vi "DMM DCVM Immediate Trigger Delay.vi"() -> ()   [LabVIEW 2021]
uses:
  DMM_DC-RMS Voltage Measurement/Typedefs/Function Settings.ctl
  <instrlib>/niDMM/nidmm.llb/niDMM Resolution in Digits.ctl
  DMM_DC-RMS Voltage Measurement/Typedefs/Timing & Trigger Settings.ctl
  <instrlib>/niDMM/nidmm.llb/niDMM Trigger.ctl
  <instrlib>/niDMM/nidmm.llb/niDMM Slope.ctl
  DMM_DC-RMS Voltage Measurement/Typedefs/Measurement.ctl
  DMM Mixed Measurements/DMM Mixed Meas Typedefs/DMM Execution Settings.ctl
  Signal Voltage Generation/Typedefs/Signal Generation Settings.ctl
  Signal Voltage Generation/Typedefs/Generation Types.ctl
  Signal Voltage Generation/Typedefs/Single Tone Settings.ctl
  Signal Voltage Generation/Typedefs/Waveform Type.ctl
  Signal Voltage Generation/Typedefs/Tone Settings.ctl
  Common/Typedefs/Execution Options - Measure.ctl
  DMM_DC-RMS Voltage Measurement/DMM_DC-RMS Voltage Measurement.lvlib
  Signal Voltage Generation/DAQ_Signal Voltage Generation.lvlib
  DMM Mixed Measurements/DMM_Mixed Measurement.lvlib
panel:
  in  "Signal Generation Settings":T1={"Generation Type"=enum."Single Tone", "Generation Time (s)"=4.0, "Voltage Offset (v)"=0.0, "Single Tone Settings"={"Waveform Type"=enum."Sine Wave", "Frequency (Hz)"=100.0, "Amplitude (V)"=1.0, "Duty Cycle (%)"=50.0}, "Multi Tone Settings"=[]} {"Voltage Offset (v)" format="%.2p"; "Generation Time (s)" format="%.2p"; "Multi Tone Settings"."Amplitude (V)" format="%.2p"; "Multi Tone Settings"."Frequency (Hz)" format="%.2p"; "Single Tone Settings"."Duty Cycle (%)" format="%.2p"; "Single Tone Settings"."Amplitude (V)" format="%.2p"; "Single Tone Settings"."Frequency (Hz)" format="%.2p"}
  out "error out":errorcluster
  out "DMM Execution Settings":T6={"Absolute\nResolution"=2.4999999999999998e-05, "Input Resistance\n(Ohm)"=1000000.0, "Digits\nResolution"=5.5, "Range"=5.0, "Minimum\nFrequency (Hz)"=40.0, "Aperture\nTime (s)"=0.1, "Auto Range\nValue"=5.0, "Settle\nTime (s)"=1.0, "Function"=2} {"Function" items=["DC Volts"=1, "AC Volts"=2, "DC Current"=3, "AC Current"=4, "2-Wire Resistance"=5, "4-Wire Resistance"=101, "Frequency"=104, "Period"=105, "AC Volts DC Coupled"=1001, "Diode"=1002, "Waveform Voltage"=1003, "Waveform Current"=1004, "Capacitance"=1005, "Inductance"=1006, "Temperature"=108]; "Absolute\nResolution" format="%#_6p"; "Input Resistance\n(Ohm)" format="%#_6p"; "Range" format="%#_6p"; "Minimum\nFrequency (Hz)" format="%#_6p"; "Aperture\nTime (s)" format="%#_6p"; "Auto Range\nValue" format="%#_6p"; "Settle\nTime (s)" format="%#_6p"}
  out "Measurement":T7={"Measured Value"=0.7067715989184996, "Out of Range"=FALSE, "Unit"="V (ac)", "Measurement"="706.772mV (ac)"} {"Measured Value" format="%^#_9e"}
  in  "Timing and Trigger Settings":T8={"AC Min Frequency (Hz)"=40.0, "Aperture Time (s)"=-1.0, "Settle Time (s)"=-1.0, "Trigger Settings"={"Trigger Delay (sec)"=2.0, "Enable Trigger?"=TRUE, "Trigger Source"=enum."Immediate", "Slope"=enum."Rising Edge"}} {"Trigger Settings"."Trigger Delay (sec)" format="%.4f"; "AC Min Frequency (Hz)" format="%.2f"}
  in  "Function Settings":T11={"Range and Function"=enum."AC 2 V", "Resolution in Digits"=5.5} {"Resolution in Digits" items=["3 1/2"=3.5, "4 1/2"=4.5, "5 1/2"=5.5, "6 1/2"=6.5, "7 1/2"=7.5]}
  in  "DMM Resource Name":refnum<k15>="DMM_4080"
  # "Frequency (Hz)"
  # "Amplitude (V)"
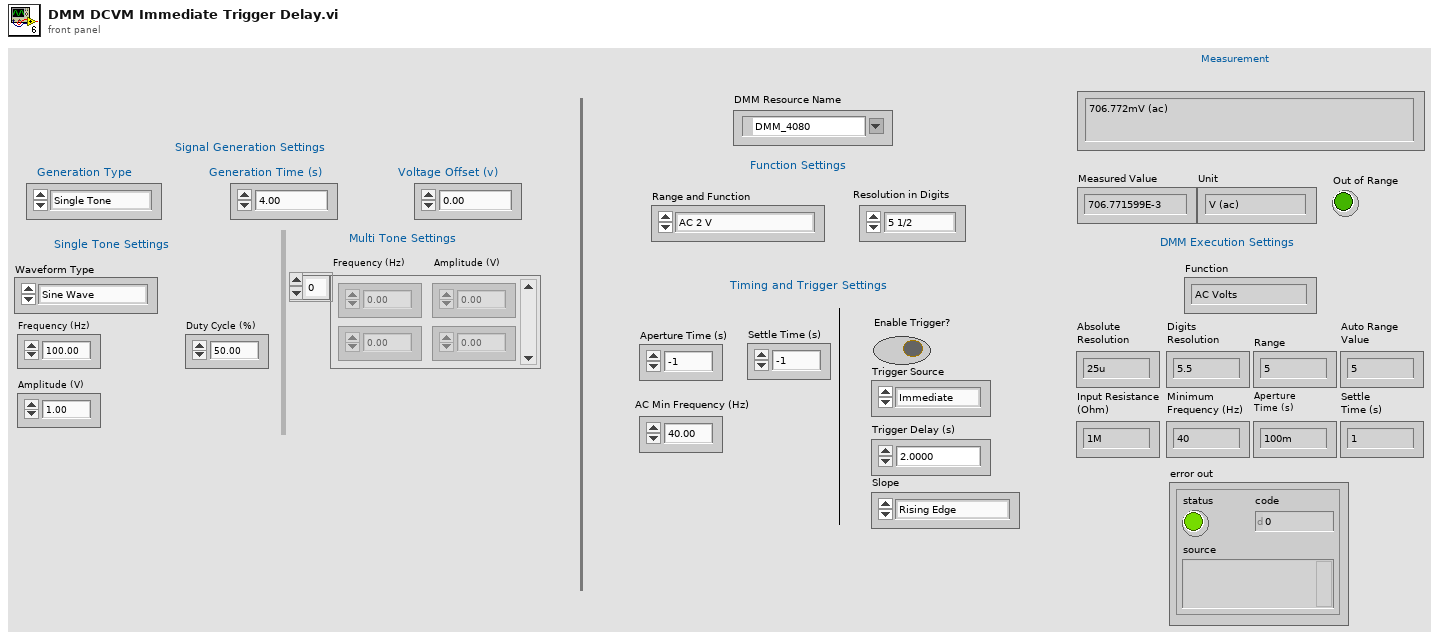
[diagram p1: front panel]
types:
  T1 = typedef "DAQ_Signal Voltage Generation.lvlib/Signal Generation Settings.ctl" = cluster{"Generation Type":T2, "Generation Time (s)":dbl, "Voltage Offset (v)":dbl, "Single Tone Settings":T3, "Multi Tone Settings":T5[]}
  T2 = typedef "DAQ_Signal Voltage Generation.lvlib/Generation Types.ctl" = enum16{"Single Tone", "Multi Tone"}
  T3 = typedef "DAQ_Signal Voltage Generation.lvlib/Single Tone Settings.ctl" = cluster{"Waveform Type":T4, "Frequency (Hz)":dbl, "Amplitude (V)":dbl, "Duty Cycle (%)":dbl}
  T4 = typedef "DAQ_Signal Voltage Generation.lvlib/Waveform Type.ctl" = enum16{"Sine Wave", "Square Wave"}
  T5 = typedef "DAQ_Signal Voltage Generation.lvlib/Tone Settings.ctl" = cluster{"Frequency (Hz)":dbl, "Amplitude (V)":dbl}
  T6 = typedef "DMM_Mixed Measurement.lvlib/DMM Execution Settings.ctl" = cluster{"Absolute\nResolution":dbl, "Input Resistance\n(Ohm)":dbl, "Digits\nResolution":dbl, "Range":dbl, "Minimum\nFrequency (Hz)":dbl, "Aperture\nTime (s)":dbl, "Auto Range\nValue":dbl, "Settle\nTime (s)":dbl, "Function":i32}
  T7 = typedef "DMM_DC-RMS Voltage Measurement.lvlib/Measurement.ctl" = cluster{"Measured Value":dbl, "Out of Range":bool, "Unit":string, "Measurement":string}
  T8 = typedef "DMM_DC-RMS Voltage Measurement.lvlib/Timing & Trigger Settings.ctl" = cluster{"AC Min Frequency (Hz)":dbl, "Aperture Time (s)":dbl, "Settle Time (s)":dbl, "Trigger Settings":cluster{"Trigger Delay (sec)":dbl, "Enable Trigger?":bool, "Trigger Source":T9, "Slope":T10}}
  T9 = typedef "niDMM Trigger.ctl" = enum16{"Immediate", "External", "TTL 0", "TTL 1", "TTL 2", "TTL 3", "TTL 4", "TTL 5", "TTL 6", "Software", "TTL 7", "PXI Star", "LBR Trig 1", "Aux Trig 1"}
  T10 = typedef "niDMM Slope.ctl" = enum16{"Rising Edge", "Falling Edge"}
  T11 = typedef "DMM_DC-RMS Voltage Measurement.lvlib/Function Settings.ctl" = cluster{"Range and Function":enum16{"DC Voltage Auto Range", "DC 100 mV", "DC 1 V ", "DC 10 V", "DC 100 V", "DC 300 V", " ", "AC Voltage Auto Range", "AC 50 mV", "AC 200 mV", "AC 500 mV", "AC 2 V", "AC 5 V", "AC 20 V", "AC 50 V", "AC 300 V"}, "Resolution in Digits":T12}
  T12 = typedef "niDMM Resolution in Digits.ctl" = dbl
  T13 = typedef "Execution Options - Measure.ctl" = enum16{"Configure & Measure", "Configure only", "Measure only"}
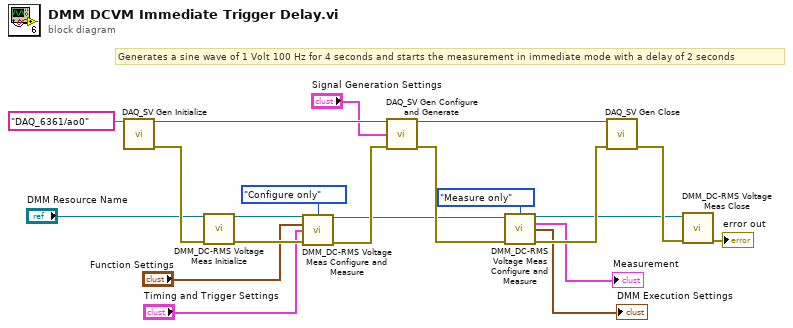
[diagram p0: block diagram]
diagram:
  # "Generates a sine wave of 1 Volt 100 Hz for 4 seconds and starts the measurement in immediate mode with a delay of 2 seconds"
  n1 = call "DAQ_SV Gen Initialize.vi"("Physical Channels"=tag "DAQ_6361/ao0") -> ("DAQmx Task Out"=w20:refnum<k21>, "error out"=w21:errorcluster)  [unwired: 13 in]
  n2 = call "DMM_DC-RMS Voltage Meas Initialize.vi"("DMM Resource Name"="DMM Resource Name", "error in"=w21) -> ("DMM Handle Out"=w11:refnum<k15>, "error out"=w18:errorcluster)  [unwired: 12 in]
  n3 = call "DMM_DC-RMS Voltage Meas Configure and Measure.vi"("DMM Handle In"=w11, "Execution Option"=Execution_Options_-_Measure."Configure only", "Function Settings"="Function Settings", "Timing and Trigger Settings"="Timing and Trigger Settings", "error in"=w18) -> ("DMM Handle Out"=w10:refnum<k15>, "error out"=w17:errorcluster)  [unwired: 7 in, 2 out]
  n4 = call "DAQ_SV Gen Configure and Generate.vi"("DAQmx Task In"=w20, "Signal Generation Settings"="Signal Generation Settings", "error in"=w17) -> ("DAQmx Task Out"=w19:refnum<k21>, "error out"=w16:errorcluster)  [unwired: 10 in, 1 out]
  n5 = call "DMM_DC-RMS Voltage Meas Configure and Measure.vi"("DMM Handle In"=w10, "Execution Option"=Execution_Options_-_Measure."Measure only", "error in"=w16) -> ("DMM Handle Out"=w9:refnum<k15>, "Measurement"=→"Measurement":T7, "DMM Execution Settings"=→"DMM Execution Settings":T6, "error out"=w15:errorcluster)  [unwired: 9 in]
  n6 = call "DAQ_SV Gen Close.vi"("DAQmx Task In"=w19, "error in"=w15) -> ("error out"=w14:errorcluster)  [unwired: 13 in]
  n7 = call "DMM_DC-RMS Voltage Meas Close.vi"("DMM Handle In"=w9, "error in"=w14) -> ("error out"=→"error out":errorcluster)  [unwired: 13 in]
